vi "Run Working Thread.vi"(8 "error in (no error)":errorcluster) -> (0 "error out":errorcluster)   [LabVIEW 2017, in "WebServiceImporter.lvlib" / "Main Panel.lvlib" / "Progress.lvlib"]
uses:
  <vilib>/Platform/WebService/Main Panel/Pages/Progress/Progress.lvlib
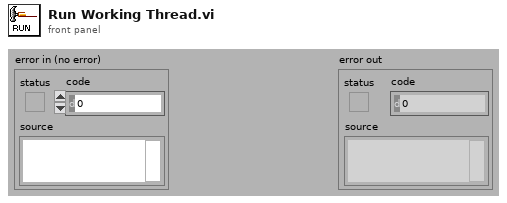
[diagram p1: front panel]
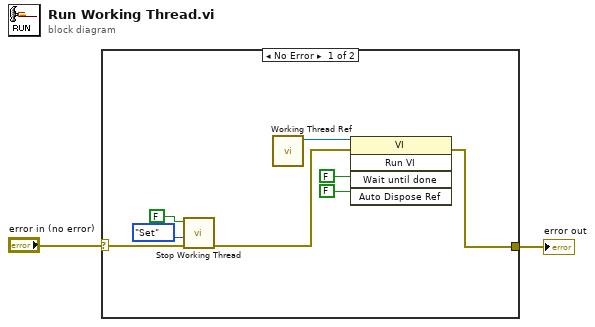
[diagram p0: block diagram]
diagram:
  n1 = case shown="No Error" "error in (no error)" {
    selector: "error in (no error)" -> [w4 w11]
    tunnel: [w10 w11] -> w1
    frame No Error {
      n2 = call <vilib>:"Stop Working Thread.vi"("error in (no error)"=w4, "Operation"=enum16{"Get", "Set"}."Set", "Stop the working thread"=FALSE) -> ("error out"=w3:errorcluster)  [unwired: 7 in, 1 out]
      n3 = call <vilib>:"Working Thread Ref.vi"() -> ("VI Refnum (out)"=w7:refnum<vi>)  [unwired: 10 in, 1 out]
      n4 = invoke class="VI" method="Run VI"(reference=w7, error in=w3, "Wait until done"=FALSE ("Wait Until Done"), "Auto Dispose Ref"=FALSE ("Auto Dispose Reference")) -> (error out=w10:errorcluster)  [unwired: 1 in, 4 out]
    }
    frame Error {
    }
  }
  "error out" <- w1
